vi "Send Response.vi"(8 "error in (no error)":errorcluster, 9 "timeout in ms (0)":i32 format="%d ms", 10 "response":T1, 11 "Transceiver Thread in":refnum<class "Transceiver Thread.lvclass">) -> (0 "error out":errorcluster, 1 "timed out?":bool, 3 "Transceiver Thread out":refnum<class "Transceiver Thread.lvclass">)   [LabVIEW 2017, in "Data Sharing Framework Engine.lvlib" / "Transceiver Thread.lvclass"]
uses:
  Transceiver Thread.lvclass
  Interfaces/Transceiver Interface/Response Data.ctl
  Interfaces/Transceiver Interface/Response.ctl
  Interfaces/Transceiver Interface/Response Parameters.ctl
  Transceiver Thread.lvclass/Transceiver Thread.ctl
  Interfaces/Transceiver Interface/Write Transceiver Response.vi
  Interfaces/Transceiver Interface/Transceiver Interface.lvclass
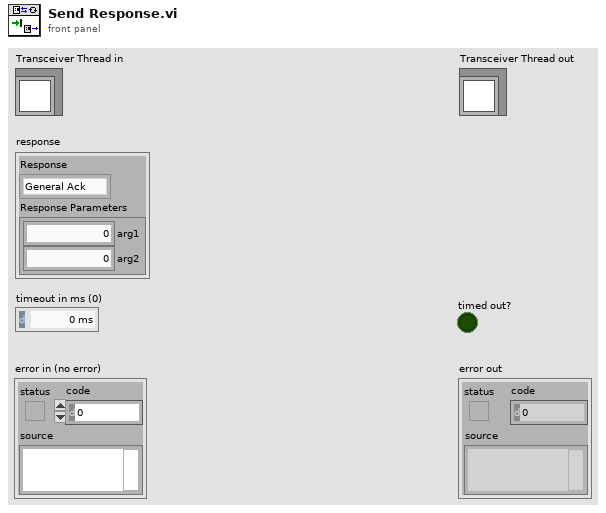
[diagram p1: front panel]
types:
  T1 = typedef "Data Sharing Framework Engine.lvlib/Transceiver Interface.lvclass/Response Data.ctl" = cluster{"Response":T2, "Response Parameters":T3}
  T2 = typedef "Data Sharing Framework Engine.lvlib/Transceiver Interface.lvclass/Response.ctl" = enum8{"General Ack", "Shutting Down"}
  T3 = typedef "Data Sharing Framework Engine.lvlib/Transceiver Interface.lvclass/Response Parameters.ctl" = cluster{"arg1":u64, "arg2":u64}
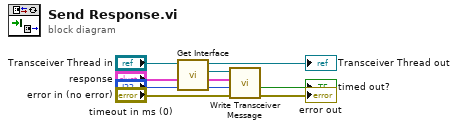
[diagram p0: block diagram]
diagram:
  n1 = call "Get Interface.vi"("Transceiver Thread in"="Transceiver Thread in") -> ("Interface"=w7:refnum<class "Transceiver Interface.lvclass">, "Transceiver Thread out"=→"Transceiver Thread out":refnum<class "Transceiver Thread.lvclass">)  [unwired: 9 in]
  n2 = call-poly "Write Transceiver Message.vi"("error in (no error)"="error in (no error)", "timeout in ms (0)"="timeout in ms (0)", "response"="response", "Transceiver Interface in"=w7) -> ("error out"=→"error out":errorcluster, "timed out?"=→"timed out?":bool)  [unwired: 5 in, 1 out]
